vi "vPage_9234+9205_hammer.vi"() -> ()   [LabVIEW 2022 SP3]
uses:
  <vilib>/Utility/sysdir.llb/System Directory Type.ctl
  <vilib>/express/express analysis/Spectral/Block/exnSpectralBlock spectral measurements RMS poly.vi
  <vilib>/express/express analysis/Spectral/Block/exnSpectralBlock spectral measurements RMS DDT.vi
  <vilib>/express/express analysis/Spectral/XNode/ExpressSpectralMeasurementsBlockNode.xnode
panel:
  out "DAQ":i32
  in  "Show":bool
  in  "¸ê®Æ§¨\nµù°O>":string
  out "DAQ Stoped":bool
  in  "Sample \nto Read":i32=25600
  in  "Sample\nRate":dbl=25600.0
  in  "Enable Saving":bool
  in  "Stop":bool
  out "C1-Save":bool
  out "C1-Trigger":bool
  out "C1-All":dynamicdata(graph)
  out "C1-0":dynamicdata(graph)
  out "C1-0 2":dynamicdata(graph)
  out "C1-0 3":dynamicdata(graph)
  # "使用前請先確認 \nDAQ 擷取卡設定"
  # "本頁畫面顯示為 觸發後訊號"
  # "FFT Filter by useing High-pass with Lower Cut-Off (Hz)"
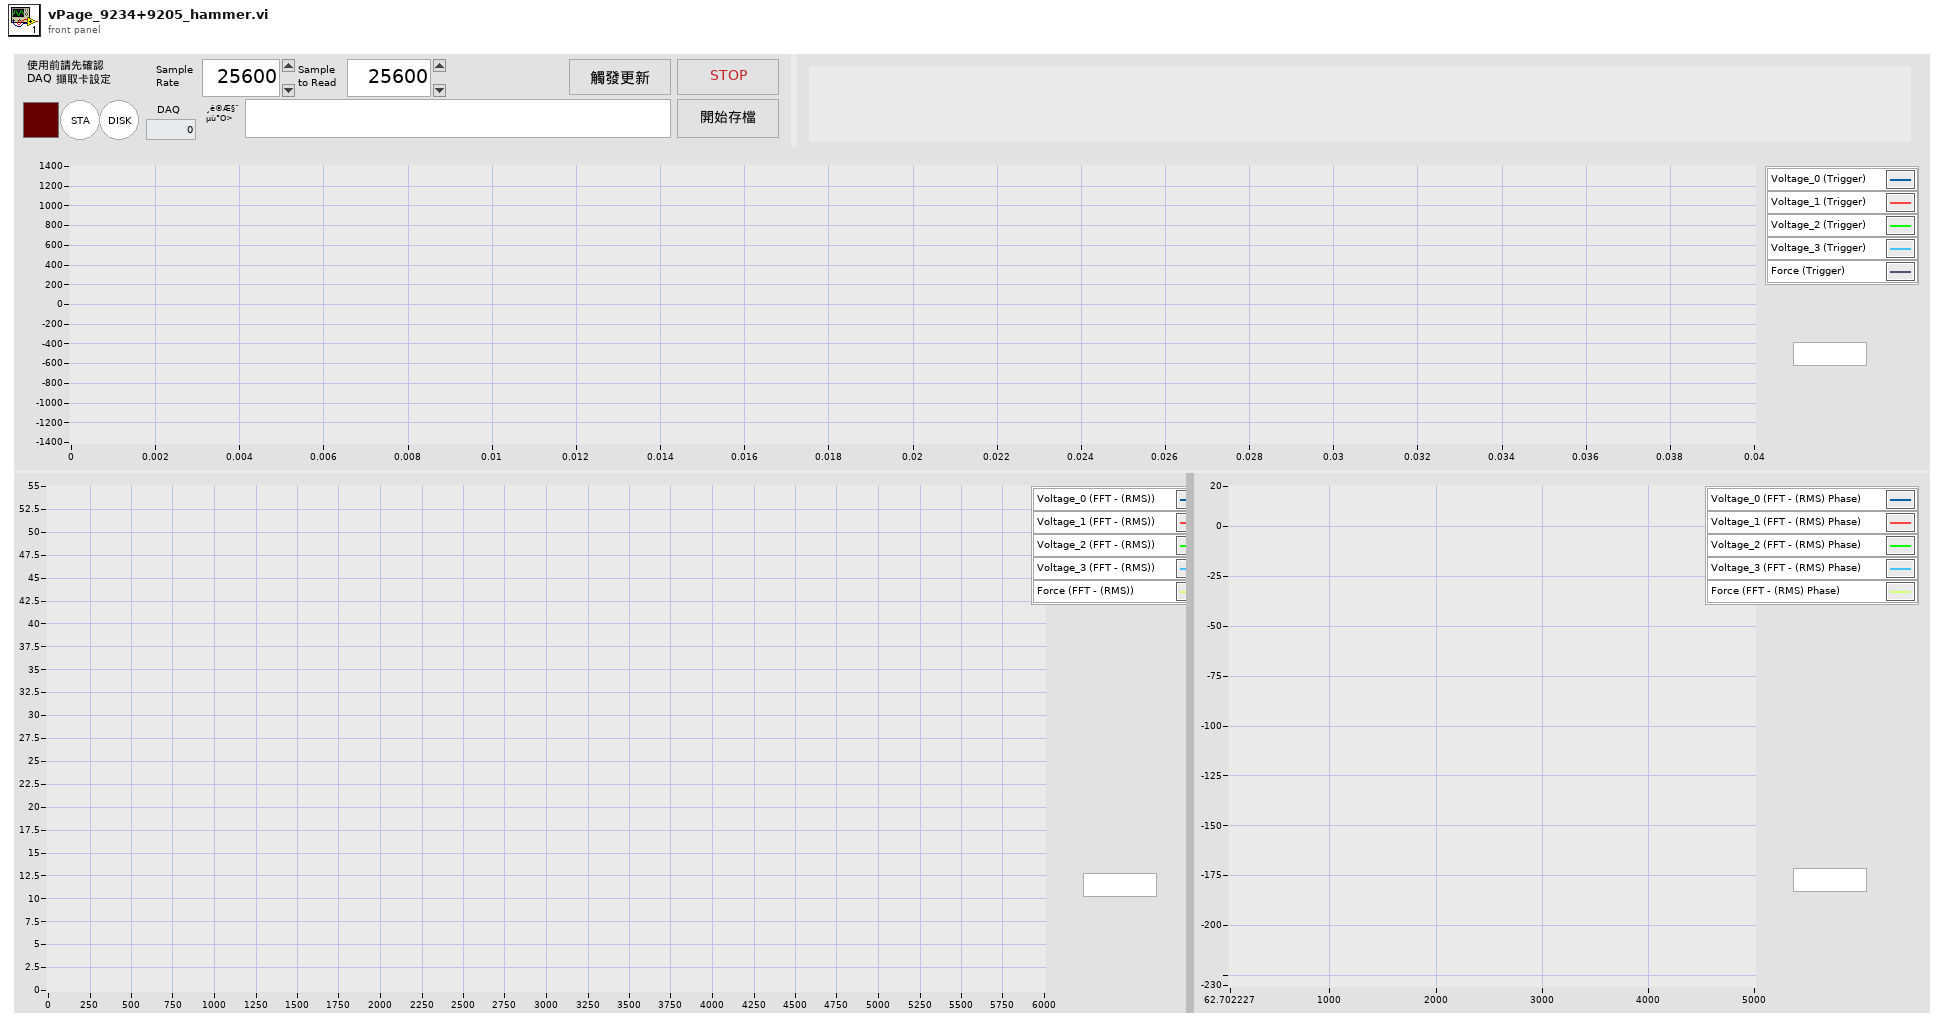
[diagram p1: front panel]
types:
  T1 = enum8{"Enabled", "Disabled", "Disabled and Grayed Out"}
  T2 = typedef "System Directory Type.ctl" = i32
  T3 = cluster{"task out":refnum<k21>, "data":dynamicdata}
  T4 = cluster{"averaging mode":u16, "weighting mode":u16, "number of averages":u32}
  T5 = cluster{"dB On (F)":bool, "unwrap phase (F)":bool, "convert to degree (F)":bool}
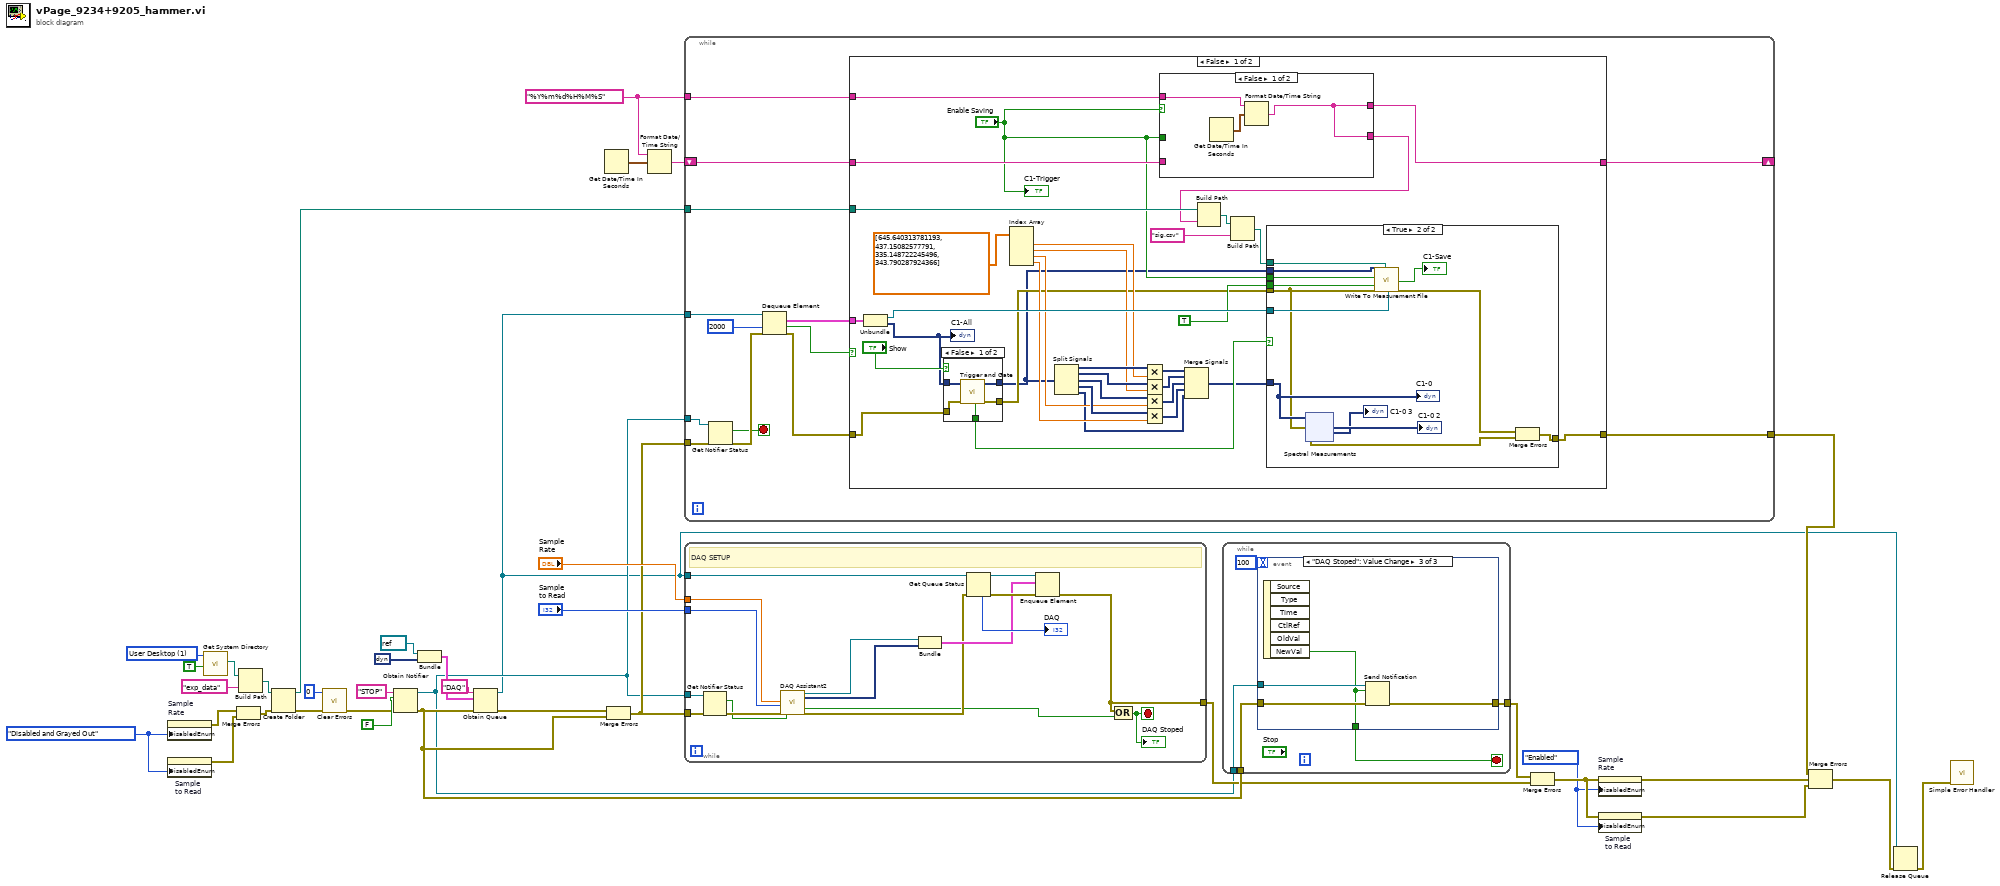
[diagram p0: block diagram]
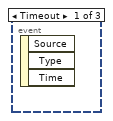
[diagram p2: hidden frame]
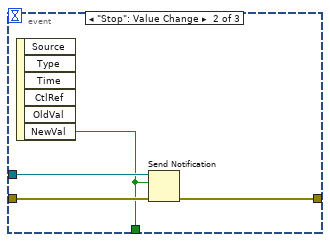
[diagram p3: hidden frame]
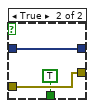
[diagram p4: hidden frame]
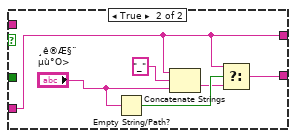
[diagram p6: hidden frame]
diagram:
  w7 = T1."Enabled" ("Disabled")
  w12 = T1."Disabled and Grayed Out" ("Disabled")
  w13 = "%Y%m%d%H%M%S" ("time format string (%c)")
  w23 = T2 1 items=["User Home"=0, "User Desktop"=1, "User Documents"=2, "User Application Data"=3, "User Preferences"=4, "User Temporary"=5, "Public Documents"=6, "Public Application Data"=7, "Public Preferences"=8, "Public Cache"=13, "System Core Libraries"=9, "System Installed Libraries"=10, "Application Files"=11, "Boot Volume Root"=12] ("system directory type")
  n1 = property on="Sample\nRate" class="DigNum (strict)"("DisabledEnum"=w12) -> (error out=w11:errorcluster)  [unwired: 2 in, 1 out]
  n2 = property on="Sample \nto Read" class="DigNum (strict)"("DisabledEnum"=w12) -> (error out=w9:errorcluster)  [unwired: 2 in, 1 out]
  n3 = call <vilib>:"Get System Directory.vi"("create directory if not found? (F)"=TRUE, "system directory type"=w23) -> ("system directory"=w25:path)  [unwired: 9 in]
  n4 = Merge Errors(w11, w9) -> (w10:errorcluster)
  n5 = Build Path(base path=w25, name or relative path="exp_data") -> (appended path=w19:path)
  n6 = Create Folder(path (use dialog)=w19, error in=w10) -> (created path=w18:path, error out=w21:errorcluster)  [unwired: 1 in, 1 out]
  n7 = call <vilib>:"Clear Errors.vi"("error in (no error)"=w21, "specific error code to clear (0: all)"=0) -> ("error out"=w20:errorcluster)  [unwired: 4 in, 1 out]
  n8 = Obtain Notifier(name (unnamed)="STOP", notification data type=FALSE, error in (no error)=w20) -> (notifier out=w14:refnum<notifier>, error out=w17:errorcluster)  [unwired: 1 in, 1 out]
  n9 = Bundle("task out"=refnum<k21> refnum, "data"=dynamicdata []) -> (w30:T3)  [unwired: 1 in]
  n10 = Obtain Queue(name (unnamed)="DAQ", element data type=w30, error in (no error)=w17) -> (queue out=w1:refnum<queue>, error out=w38:errorcluster)  [unwired: 2 in, 1 out]
  n11 = Get Date/Time In Seconds() -> (seconds since 1Jan1904=w28:timestamp)
  n12 = Merge Errors(w38, w17) -> (w29:errorcluster)
  n13 = Format Date/Time String(time format string (%c)=w13, seconds (now)=w28) -> (date/time string=w27:string)  [unwired: 1 in]
  n14 = while {
    tunnel: w29 -> [w52]
    tunnel: w14 -> [w50]
    tunnel: w1 -> [w49]
    shift-right: [w39] -> _
    shift-left: w27 -> [w43]
    tunnel: w18 -> [w44]
    tunnel: [w40] -> w2
    tunnel: w13 -> [w42]
    stop <- w47 stop-if-true
    n15 = Get Notifier Status(notifier=w50, error in (no error)=w52) -> (current notification=w47:bool, error out=w51:errorcluster)  [unwired: 3 out]
    n16 = Dequeue Element(queue=w49, timeout in ms (-1)=2000, error in (no error)=w51) -> (element=w45:T3, timed out?=w46:bool, error out=w41:errorcluster)  [unwired: 1 out]
    n17 = case shown="False" w46 {
      tunnel: w45 -> [w86 _]
      tunnel: w41 -> [w59 w128]
      tunnel: w43 -> [w84 w129]
      tunnel: [w83 w129] -> w39
      tunnel: w44 -> [w82 _]
      tunnel: [w57 w128] -> w40
      tunnel: w42 -> [w76 _]
      frame False {
        n18 = Unbundle(w86) -> ("task out"=w85:refnum<k21>, "data"=w54:dynamicdata)
        "C1-All" <- w54
        n19 = case shown="False" "Show" {
          tunnel: [w91 TRUE ("Data Available")] -> w60
          tunnel: w54 -> [w90 w94]
          tunnel: [w89 w94] -> w53
          tunnel: w59 -> [w88 w93]
          tunnel: [w87 w93] -> w58
          frame False {
            n20 = call "Trigger and Gate"("error in (no error)"=w88, "Signals"=w90) -> ("error out"=w87:errorcluster, "Triggered Signals"=w89:dynamicdata, "Data Available"=w91:bool)  [unwired: 6 in, 1 out]
          }
          frame True {
          }
        }
        n21 = Index Array(array=dbl[] [645.640313781193, 437.15082577791, 335.148722245496, 343.790287924366]) -> (element #1=w72:dbl, element #2=w68:dbl, element #3=w67:dbl, element #4=w66:dbl)  [unwired: 4 in]
        n22 = Split Signals(w53) -> (w74:dynamicdata, w71:dynamicdata, w70:dynamicdata, w69:dynamicdata, w61:dynamicdata)  [unwired: 5 in]
        n23 = Multiply(x=w74, y=w72) -> (x*y=w62:dynamicdata)
        n24 = Multiply(x=w71, y=w68) -> (x*y=w63:dynamicdata)
        n25 = Multiply(x=w70, y=w67) -> (x*y=w64:dynamicdata)
        n26 = Multiply(x=w69, y=w66) -> (x*y=w65:dynamicdata)
        n27 = case shown="False" "Enable Saving" {
          tunnel: [w119 w123] -> w83
          tunnel: "Enable Saving" -> [_ _]
          tunnel: w84 -> [_ w123]
          tunnel: [w119 w125] -> w77
          tunnel: w76 -> [w120 _]
          frame False {
            n28 = Get Date/Time In Seconds() -> (seconds since 1Jan1904=w121:timestamp)
            n29 = Format Date/Time String(time format string (%c)=w120, seconds (now)=w121) -> (date/time string=w119:string)  [unwired: 1 in]
          }
          frame True {
            n30 = Empty String/Path?(string/path="¸ê®Æ§¨\nµù°O>") -> (empty?=w127:bool)
            n31 = Concatenate Strings(w123, "_" ("string"), "¸ê®Æ§¨\nµù°O>") -> (w126:string)
            n32 = Select(t=w123, s=w127, f=w126) -> (s? t:f=w125:string)
          }
        }
        n33 = Merge Signals(w62, w63, w64, w65, w61) -> (w55:dynamicdata)
        n34 = Build Path(base path=w82, name or relative path=w77) -> (appended path=w81:path)
        n35 = Build Path(base path=w81, name or relative path="sig.csv") -> (appended path=w79:path)
        n36 = case shown="True" w60 {
          tunnel: w58 -> [w95 w101]
          tunnel: w85 -> [_ w108]
          tunnel: w79 -> [_ w107]
          tunnel: TRUE ("new_file") -> [_ w106]
          tunnel: "Enable Saving" -> [_ w104]
          tunnel: w55 -> [_ w102]
          tunnel: [w95 w98] -> w57
          tunnel: w53 -> [_ w96]
          frame False {
          }
          frame True {
            n37 = xnode ("Spectral Measurements")("Signals"=w102, "error in (no error)"=w101) -> ("FFT - (RMS)"=→"C1-0 2":dynamicdata, "Phase"=→"C1-0 3":dynamicdata, "error out"=w99:errorcluster)
            n38 = call "Write To Measurement File"("Signals"=w96, "Enable"=w104, "new_file"=w106, "error in (no error)"=w101, "Filename"=w107, "DAQmx Task"=w108) -> ("Saving Data"=→"C1-Save":bool, "error out"=w100:errorcluster)  [unwired: 11 in, 1 out]
            n39 = Merge Errors(w100, w99) -> (w98:errorcluster)
            "C1-0" <- w102
          }
        }
        "C1-Trigger" <- "Enable Saving"
      }
      frame True {
      }
    }
  }
  n40 = while {
    tunnel: [w145] -> w15
    tunnel: w1 -> [w142]
    tunnel: w29 -> [w141]
    tunnel: w14 -> [w140]
    tunnel: "Sample \nto Read" -> [w134]
    tunnel: "Sample\nRate" -> [w135]
    stop <- w143 stop-if-true
    # "DAQ SETUP"
    n41 = Get Notifier Status(notifier=w140, error in (no error)=w141) -> (current notification=w133:bool, error out=w137:errorcluster)  [unwired: 3 out]
    n42 = call "DAQ Assistant2"("rate"=w135, "number of samples"=w134, "error in"=w137, "stop (F)"=w133) -> ("task out"=w131:refnum<k21>, "data"=w130:dynamicdata, "stopped"=w132:bool, "error out"=w136:errorcluster)  [unwired: 12 in]
    n43 = Bundle("task out"=w131, "data"=w130) -> (w138:T3)  [unwired: 1 in]
    n44 = Get Queue Status(queue=w142, error in (no error)=w136) -> (queue out=w139:refnum<queue>, error out=w146:errorcluster, # elements in queue=→"DAQ":i32)  [unwired: 1 in, 5 out]
    n45 = Enqueue Element(queue=w139, element=w138, error in (no error)=w146) -> (error out=w145:errorcluster)  [unwired: 1 in, 2 out]
    n46 = Compound Arithmetic op=OR(w145, w132) -> (w143:bool)
    "DAQ Stoped" <- w143
  }
  n47 = while {
    tunnel: w17 -> [w151]
    tunnel: [w150] -> w16
    tunnel: w14 -> [w149]
    stop <- w148 stop-if-true
    n48 = event shown="[2] \"DAQ Stoped\": Value Change" {
      selector: _ -> [_ _ _]
      dyn-events: _ -> [_ _ _]
      timeout: 100 -> [_ _ _]
      tunnel: w151 -> [_ w155 w159]
      tunnel: [_ w154 w158] -> w150
      tunnel: w149 -> [_ w153 w157]
      tunnel: [_ w152 w156] -> w148
      event Timeout {
        n49 = event-data() -> ()  [unwired: 1 in, 3 out]
      }
      event "Stop": Value Change {
        n50 = event-data() -> ("NewVal"=w152:bool)  [unwired: 1 in, 5 out]
        n51 = Send Notification(notification=w152, notifier=w153, error in (no error)=w155) -> (error out=w154:errorcluster)  [unwired: 1 out]
      }
      event "DAQ Stoped": Value Change {
        n52 = event-data() -> ("NewVal"=w156:bool)  [unwired: 1 in, 5 out]
        n53 = Send Notification(notification=w156, notifier=w157, error in (no error)=w159) -> (error out=w158:errorcluster)  [unwired: 1 out]
      }
    }
  }
  n54 = Merge Errors(w16, w15) -> (w8:errorcluster)
  n55 = property on="Sample\nRate" class="DigNum (strict)"(error in=w8, "DisabledEnum"=w7) -> (error out=w6:errorcluster)  [unwired: 1 in, 1 out]
  n56 = property on="Sample \nto Read" class="DigNum (strict)"(error in=w8, "DisabledEnum"=w7) -> (error out=w5:errorcluster)  [unwired: 1 in, 1 out]
  n57 = Merge Errors(w2, w6, w5) -> (w3:errorcluster)
  n58 = Release Queue(queue=w1, error in (no error)=w3) -> (error out=w4:errorcluster)  [unwired: 1 in, 2 out]
  n59 = call <vilib>:"Simple Error Handler.vi"("error in (no error)"=w4) -> ()  [unwired: 4 in, 5 out]
